vi "dispatch.vi"(8 "error in (no error)":errorcluster, 10 "Parameters in":refnum<class "IBaseObject.lvclass">, 11 "IProcedure in":refnum<class "IProcedure.lvclass">) -> (0 "error out":errorcluster, 2 "Parameters out":refnum<class "IBaseObject.lvclass">, 3 "IProcedure out":refnum<class "IProcedure.lvclass">)   [LabVIEW 2022 SP3, in "openDAQ.lvlib" / "daqCoreTypes.lvlib" / "IProcedure.lvclass"]
uses:
  <instrlib>/openDAQ/Public/Classes/daqCoreTypes/IProcedure/IProcedure.lvclass
  <instrlib>/openDAQ/Public/Classes/daqCoreTypes/IProcedure/IProcedure.lvclass/IProcedure.ctl
  <instrlib>/openDAQ/Public/Classes/IBaseObject/IBaseObject.lvclass
  <instrlib>/openDAQ/Binaries/Windows/x86/copendaq32.dll
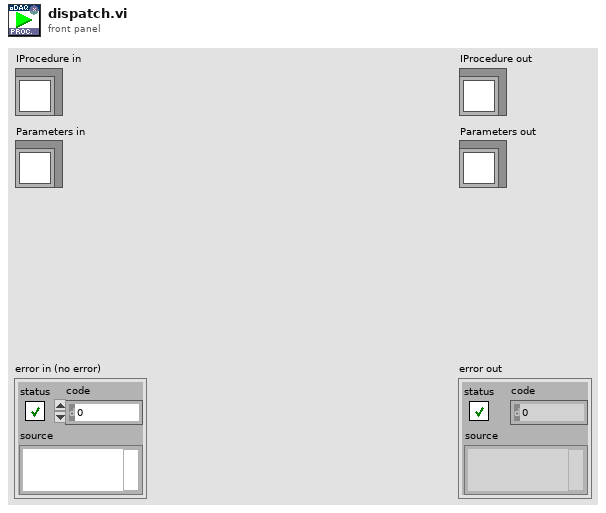
[diagram p1: front panel]
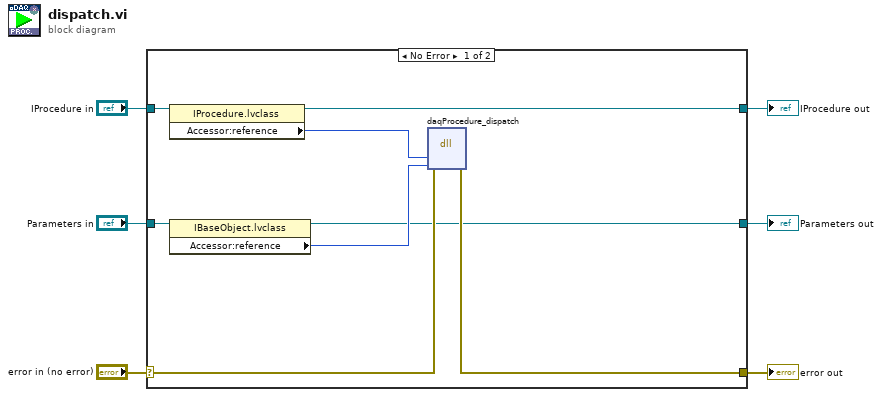
[diagram p0: block diagram]
diagram:
  n1 = case shown="No Error" "error in (no error)" {
    selector: "error in (no error)" -> [w13 w17]
    tunnel: [w12 w17] -> w5
    tunnel: [w11 w16] -> w3
    tunnel: "IProcedure in" -> [w14 w16]
    tunnel: "Parameters in" -> [w9 w15]
    tunnel: [w7 w15] -> w1
    frame No Error {
      n2 = property class="IProcedure.lvclass"(reference=w14) -> (reference out=w11:refnum<class "IProcedure.lvclass">, "Accessor:reference"=w10:i64)  [unwired: 1 in, 1 out]
      n3 = property class="IBaseObject.lvclass"(reference=w9) -> (reference out=w7:refnum<class "IBaseObject.lvclass">, "Accessor:reference"=w8:i64)  [unwired: 1 in, 1 out]
      n4 = dll-call lib="C:/Program Files (x86)/National Instruments/LabVIEW 2022/instr.lib/openDAQ/Binaries/Windows/x86/copendaq*.*" fn="daqProcedure_dispatch"(error in=w13, "procedure"=w10, "params"=w8) -> (error out=w12:errorcluster)  [unwired: 5 in, 1 out]
    }
    frame Error {
    }
  }
  "error out" <- w5
  "IProcedure out" <- w3
  "Parameters out" <- w1
